vi "Read csv teraterm configs New.vi"(8 "error in (no error)":errorcluster, 11 "Path":path=path "L:/teraterm/console_configs.csv") -> (0 "error out":errorcluster, 1 "Consoles":i32, 3 "Config name":string, 4 "Options":T1)   [LabVIEW 2013]
uses:
  Test Support VI/Tera term Serial options.ctl
panel:
  in  "Section Name":string="general"
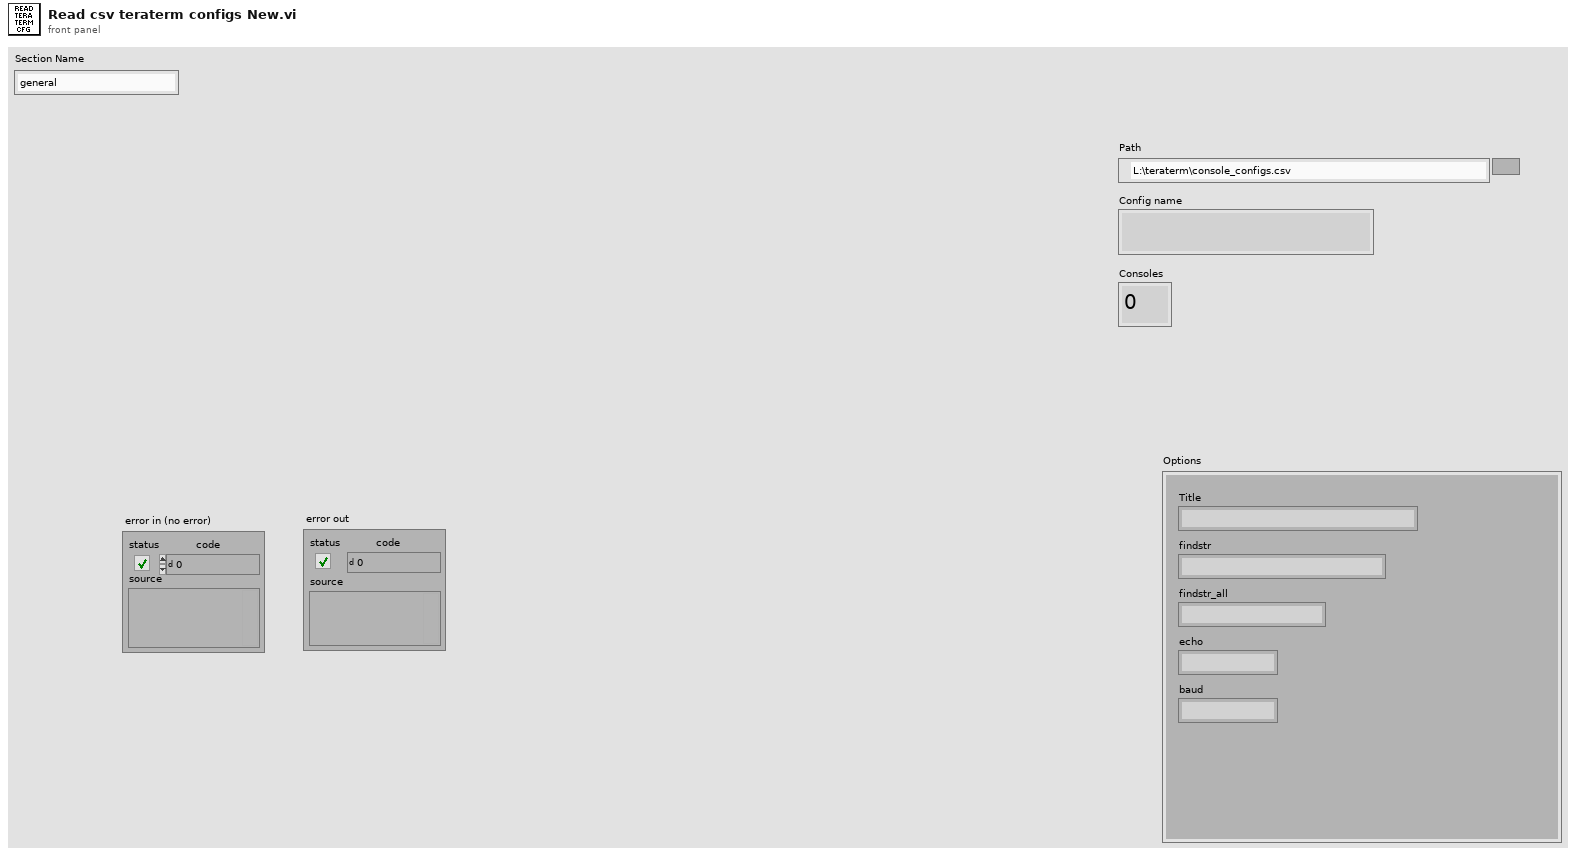
[diagram p1: front panel]
types:
  T1 = typedef "Tera term Serial options.ctl" = cluster{"Title":string, "findstr":string, "findstr_all":string, "echo":string, "baud":string}
  T2 = cluster{"Title":string, "findstr":string, "findstr_all":string, "echo":string, "baud":string}
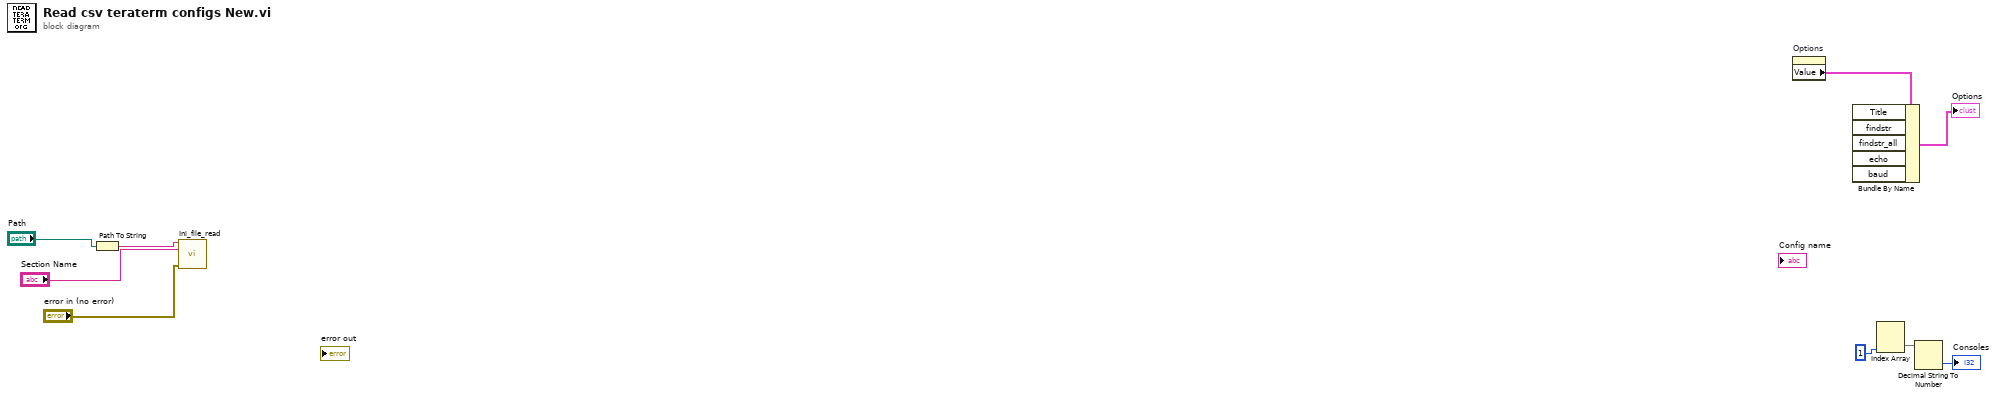
[diagram p0: block diagram]
diagram:
  n1 = Path To String(path="Path") -> (string=w3:string)
  n2 = call "Ini_file_read.vi"("Config file path name"=w3, "Section Name"="Section Name", "error in (no error)"="error in (no error)") -> ()  [unwired: 9 in, 4 out]
  n3 = property on="Options" class="Clust (strict)"() -> ("Value"=w12:T2)  [unwired: 2 in, 2 out]
  n4 = Bundle By Name(cluster=w12) -> (→"Options":T2, "Title"=w11:string, "findstr"=w10:string, "findstr_all"=w9:string, "echo"=w8:string, "baud"=w7:string)
  n5 = Index Array(index (col)=1 ("disabled index (col)")) -> (array=w5:string[][], element=w15, index (row)=w13:i32)
  n6 = Decimal String To Number(string=w15) -> (number=→"Consoles":i32)  [unwired: 2 in, 1 out]
